vi "AddTwoNumbersInClusterArray.vi"(3 "Numeric 2":dbl, 4 "Numeric 1":dbl, 5 "Array In":cluster{".NET Refnum":refnum<k24>}[](array[cluster])) -> (0 "error out":errorcluster, 1 "Sum":dbl, 2 "Array Out":cluster{".NET Refnum":refnum<k24>}[](array[cluster]))   [LabVIEW 2012]
uses:
  D:/tsdev/Tests/LVBuildValidation/12.0/Automated/FlexLVAdapter30/Refnums/DotNetRefnum/LabviewDNTest.dll
  LabviewDNTest.dll
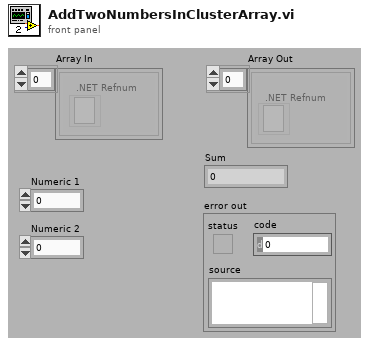
[diagram p1: front panel]
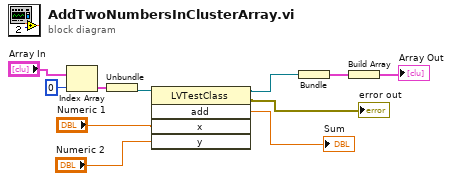
[diagram p0: block diagram]
diagram:
  n1 = Index Array(array="Array In", index=0) -> (element=w9:cluster{".NET Refnum":refnum<k24>})
  n2 = Unbundle(w9) -> (".NET Refnum"=w6:refnum<k24>)
  n3 = invoke class="LVTestClass" method="add"(reference=w6, "x"="Numeric 1", "y"="Numeric 2") -> (reference out=w5:refnum<k24>, error out=→"error out":errorcluster, "add"=→"Sum":dbl)  [unwired: 2 in, 2 out]
  n4 = Bundle(".NET Refnum"=w5) -> (w7:cluster{".NET Refnum":refnum<k24>})  [unwired: 1 in]
  n5 = Build Array(w7) -> (→"Array Out":cluster{".NET Refnum":refnum<k24>}[])
